vi "initializeStyleCollection.vi"(8 "error in (no error)":errorcluster, 11 "Document in":refnum<class "Document.lvclass">) -> (0 "error out":errorcluster, 3 "Document out":refnum<class "Document.lvclass">)   [LabVIEW 2017, in "LabVIEW NPOI.lvlib" / "Document.lvclass"]
uses:
  Document.lvclass
  Document.lvclass/Document.ctl
  Styles/Title/Title.lvclass
  C:/Users/Neo/Desktop/Dev_Tools_BR/LabVIEW_NPOI/src/Styles/Style/Style.lvclass
  Styles/Heading 1/Heading 1.lvclass
  Styles/Heading 2/Heading 2.lvclass
  Styles/Heading 3/Heading 3.lvclass
  Styles/Style/Get Style Name.vi
  Styles/Style/Style.lvclass
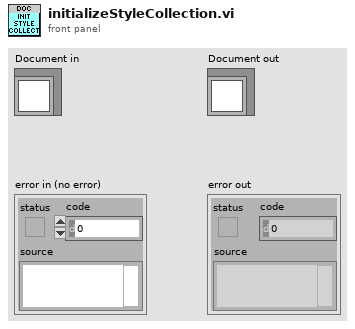
[diagram p1: front panel]
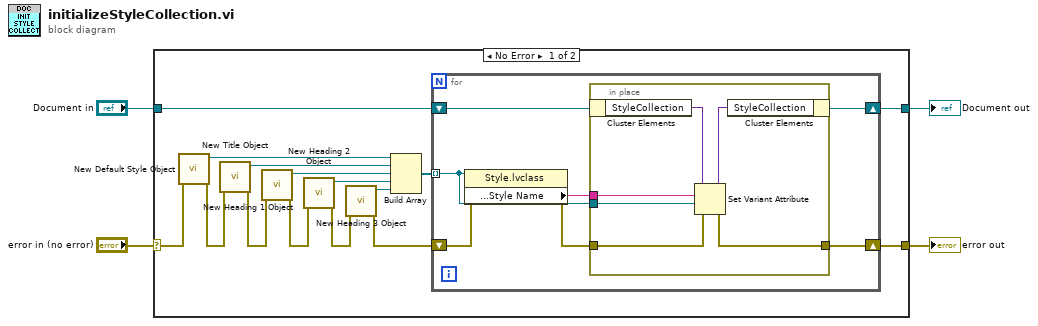
[diagram p0: block diagram]
diagram:
  n1 = case shown="No Error" "error in (no error)" {
    selector: "error in (no error)" -> [w19 w34]
    tunnel: [w6 w34] -> w3
    tunnel: [w7 w33] -> w1
    tunnel: "Document in" -> [w8 w33]
    frame No Error {
      n2 = call "New Default Style Object.vi"("error in (no error)"=w19) -> ("error out"=w18:errorcluster, "Style out"=w14:refnum<class "Style.lvclass">)  [unwired: 9 in]
      n3 = call "New Title Object.vi"("error in (no error)"=w18) -> ("error out"=w17:errorcluster, "Title out"=w13:refnum<class "Title.lvclass">)  [unwired: 9 in]
      n4 = call "New Heading 1 Object.vi"("error in (no error)"=w17) -> ("error out"=w16:errorcluster, "Heading 1 out"=w12:refnum<class "Heading 1.lvclass">)  [unwired: 9 in]
      n5 = call "New Heading 2 Object.vi"("error in (no error)"=w16) -> ("error out"=w15:errorcluster, "Heading 2 out"=w11:refnum<class "Heading 2.lvclass">)  [unwired: 9 in]
      n6 = call "New Heading 3 Object.vi"("error in (no error)"=w15) -> ("error out"=w5:errorcluster, "Heading 3 out"=w10:refnum<class "Heading 3.lvclass">)  [unwired: 9 in]
      n7 = Build Array(w14, w13, w12, w11, w10) -> (w9:refnum<class "Style.lvclass">[])
      n8 = for {
        tunnel: w9 -> [w23] mode=indexing
        shift-right: [w25] -> w7
        shift-left: w8 -> [w26]
        shift-right: [w22] -> w6
        shift-left: w5 -> [w21]
        n9 = property class="Style.lvclass"(reference=w23, error in=w21) -> (error out=w20:errorcluster, "Public VIs:Properties:Style Name"=w24:string)  [unwired: 1 out]
        n10 = in-place {
          in-place-border: w24 -> [w30]
          in-place-border: w23 -> [w29]
          in-place-border: [w28] -> w22
          in-place-border: w20 -> [w27]
          n11 = in-place-cluster #1(w26) -> ("StyleCollection"=w32:variant)
          n12 = Set Variant Attribute(Variant=w32, name=w30, value=w29, error in=w27) -> (Variant out=w31:variant, error out=w28:errorcluster)  [unwired: 1 out]
          n13 = in-place-cluster #1("StyleCollection"=w31) -> (w25:refnum<class "Document.lvclass">)
        }
      }
    }
    frame Error {
    }
  }
  "error out" <- w3
  "Document out" <- w1
